vi "ex_loop.vi"() -> ()   [LabVIEW 2012]
uses:
  <userlib>/libximc/libximc.lvlib
panel:
  out "Dif":dbl
  in  "Boolean":bool
  in  "OK Button":bool
  in  "stop":bool
  in  "WND 1":i32=1 min=1 max=8
  in  "WND 2":i32=1 min=1 max=8
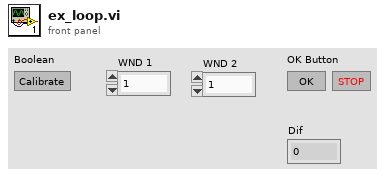
[diagram p1: front panel]
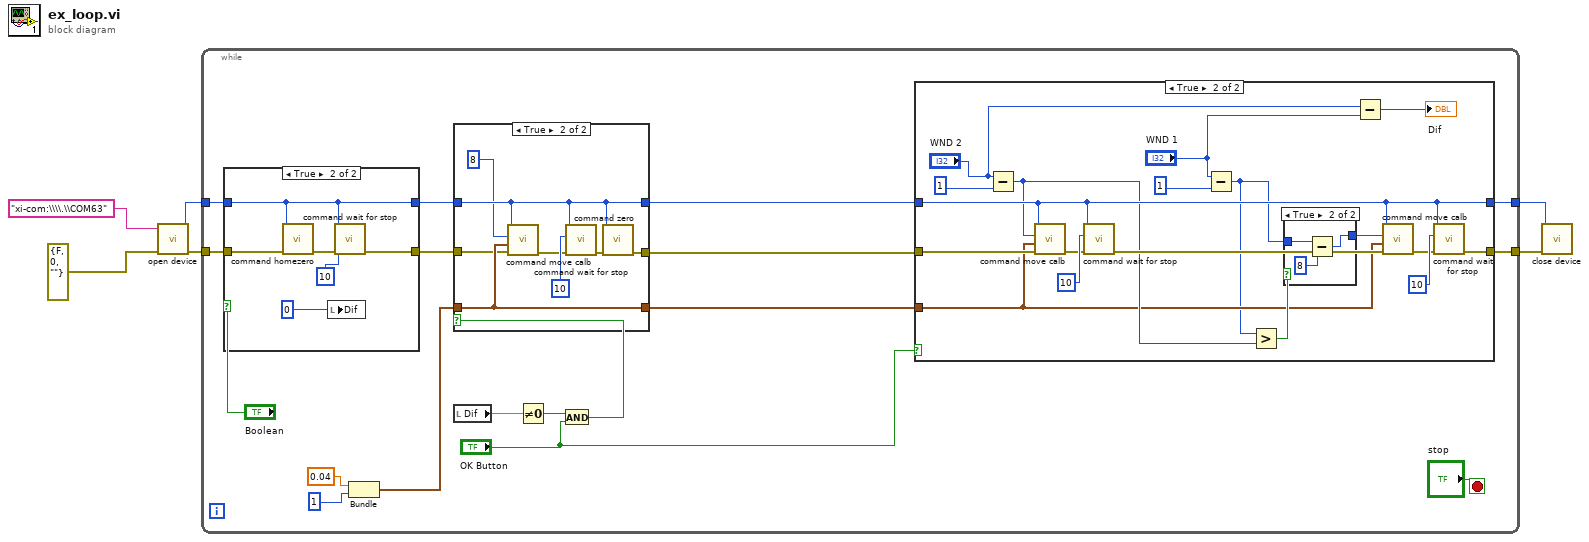
[diagram p0: block diagram]
diagram:
  n1 = call <userlib>:"open device.vi"("error in (no error)"=errorcluster {"status"=FALSE, "code"=0, "source"=""}, "uri"="xi-com:\\\\.\\COM63") -> ("error out"=w3:errorcluster, "function return"=w1:i32)  [unwired: 8 in]
  n2 = while {
    tunnel: w3 -> [w23]
    tunnel: [w22] -> w2
    tunnel: w1 -> [w18]
    tunnel: [w19] -> _
    stop <- "stop" stop-if-true
    n3 = case shown="True" "Boolean" {
      tunnel: w23 -> [w35 w42]
      tunnel: [w35 w39] -> w10
      tunnel: w18 -> [w36 w38]
      tunnel: [w36 w38] -> w11
      frame False {
      }
      frame True {
        n4 = call <userlib>:"command homezero.vi"("error in (no error)"=w42, "id"=w38) -> ("error out"=w41:errorcluster)  [unwired: 8 in, 1 out]
        n5 = local write "Dif"(0) -> ()
        n6 = call <userlib>:"command wait for stop.vi"("error in (no error)"=w41, "refresh_interval_ms"=10, "id"=w38) -> ("error out"=w39:errorcluster)  [unwired: 7 in, 1 out]
      }
    }
    n7 = Bundle(0.04, 1) -> (w8:cluster{dbl, i32})  [unwired: 1 in]
    n8 = local read "Dif"() -> (w14:dbl)
    n9 = Not Equal To 0?(x=w14) -> (x != 0?=w13:bool)
    n10 = And(x=w13, y="OK Button") -> (x .and. y?=w15:bool)
    n11 = case shown="True" w15 {
      tunnel: w11 -> [w25 w31]
      tunnel: w10 -> [w24 w28]
      tunnel: w8 -> [w26 w30]
      tunnel: [w26 w30] -> w9
      tunnel: [w25 w31] -> w7
      tunnel: [w24 w34] -> w6
      frame False {
      }
      frame True {
        n12 = call <userlib>:"command move calb.vi"("error in (no error)"=w28, "calibration"=w30, "Position"=8, "id"=w31) -> ("error out"=w29:errorcluster)  [unwired: 6 in, 1 out]
        n13 = call <userlib>:"command wait for stop.vi"("error in (no error)"=w29, "refresh_interval_ms"=10, "id"=w31) -> ("error out"=w32:errorcluster)  [unwired: 7 in, 1 out]
        n14 = call <userlib>:"command zero.vi"("error in (no error)"=w32, "id"=w31) -> ("error out"=w34:errorcluster)  [unwired: 8 in, 1 out]
      }
    }
    n15 = case shown="True" "OK Button" {
      tunnel: w6 -> [w43 w51]
      tunnel: [w43 w55] -> w22
      tunnel: w7 -> [w44 w47]
      tunnel: [w44 w47] -> w19
      tunnel: w9 -> [_ w50]
      frame False {
      }
      frame True {
        n16 = Subtract(x="WND 2", y=1) -> (x-y=w52:i32)
        n17 = call <userlib>:"command move calb.vi"("error in (no error)"=w51, "calibration"=w50, "Position"=w52, "id"=w47) -> ("error out"=w61:errorcluster)  [unwired: 6 in, 1 out]
        n18 = call <userlib>:"command wait for stop.vi"("error in (no error)"=w61, "refresh_interval_ms"=10, "id"=w47) -> ("error out"=w58:errorcluster)  [unwired: 7 in, 1 out]
        n19 = Subtract(x="WND 1", y=1) -> (x-y=w46:i32)
        n20 = Greater?(x=w46, y=w52) -> (0:w60:bool)
        n21 = case shown="True" w60 {
          tunnel: w46 -> [w63 w65]
          tunnel: [w63 w64] -> w57
          frame False {
          }
          frame True {
            n22 = Subtract(x=w65, y=8) -> (x-y=w64:i32)
          }
        }
        n23 = Subtract(x="WND 2", y="WND 1") -> (x-y=→"Dif":i32)
        n24 = call <userlib>:"command move calb.vi"("error in (no error)"=w58, "calibration"=w50, "Position"=w57, "id"=w47) -> ("error out"=w56:errorcluster)  [unwired: 6 in, 1 out]
        n25 = call <userlib>:"command wait for stop.vi"("error in (no error)"=w56, "refresh_interval_ms"=10, "id"=w47) -> ("error out"=w55:errorcluster)  [unwired: 7 in, 1 out]
      }
    }
  }
  n26 = call <userlib>:"close device.vi"("error in (no error)"=w2, "id"=w1) -> ()  [unwired: 7 in, 3 out]
